vi "Enqueue Power Spectrum.vi"(6 "plot analys?":bool, 7 "plot data?":bool, 8 "error in (no error)":errorcluster, 9 "pwr spctm":cluster{"f0":dbl, "df":dbl, "magnitude":dbl[]}, 10 "wfm dat":waveform(cdb), 11 "plot queue":refnum<queue>) -> (0 "error out":errorcluster)   [LabVIEW 2021]
uses:
  Plotting Data.ctl
  Plotting Message.ctl
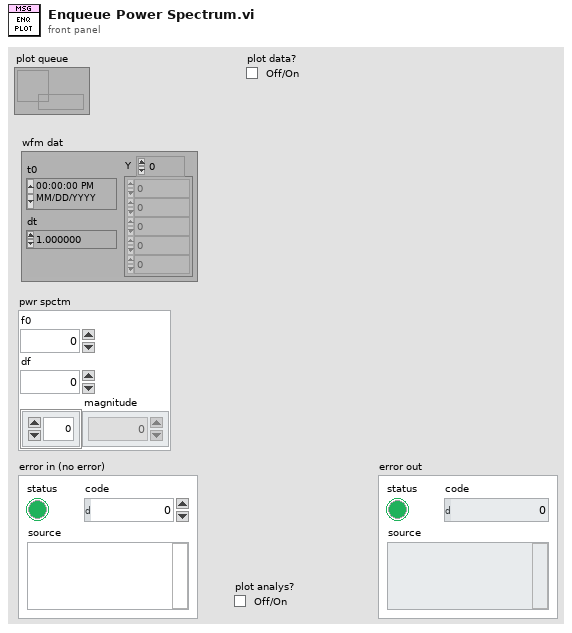
[diagram p1: front panel]
types:
  T1 = typedef "Plotting Data.ctl" = cluster{"wfm dat":waveform(cdb), "pwr sptm":cluster{"f0":dbl, "df":dbl, "magnitude":dbl[]}, "msg":T2}
  T2 = typedef "Plotting Message.ctl" = enum16{"Plot Anlalyzed Data", "Plot Acquired Data", "Exit"}
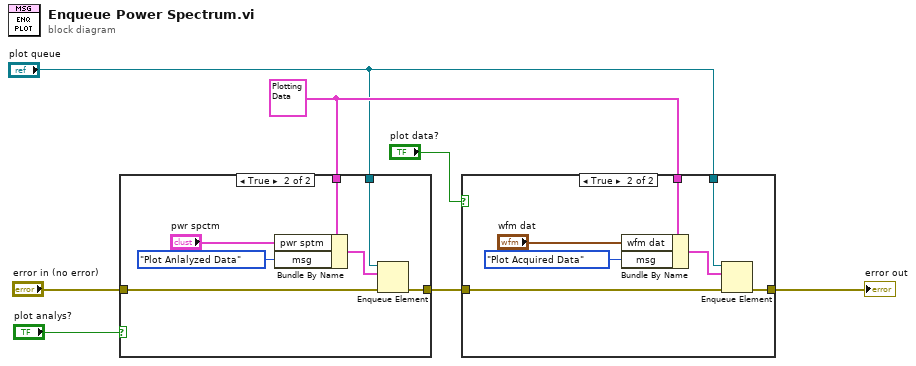
[diagram p0: block diagram]
diagram:
  w3 = T1 {"wfm dat"={"t0"=timestamp(0 s since 1904-01-01), "dt"=0.0, "Y"=[]}, "pwr sptm"={"f0"=0.0, "df"=0.0, "magnitude"=[]}, "msg"=enum."Plot Anlalyzed Data"} ("element")
  n1 = case shown="True" "plot analys?" {
    tunnel: [w8 w15] -> w4
    tunnel: "error in (no error)" -> [w8 w14]
    tunnel: "plot queue" -> [_ w13]
    tunnel: w3 -> [_ w12]
    frame False {
    }
    frame True {
      n2 = Bundle By Name(cluster=w12, "pwr sptm"="pwr spctm", "msg"=Plotting_Message."Plot Anlalyzed Data") -> (w10:T1)
      n3 = Enqueue Element(queue=w13, element=w10, error in (no error)=w14) -> (error out=w15:errorcluster)  [unwired: 1 in, 2 out]
    }
  }
  n4 = case shown="True" "plot data?" {
    tunnel: [w16 w23] -> w5
    tunnel: w4 -> [w16 w22]
    tunnel: "plot queue" -> [_ w21]
    tunnel: w3 -> [_ w20]
    frame False {
    }
    frame True {
      n5 = Bundle By Name(cluster=w20, "wfm dat"="wfm dat", "msg"=Plotting_Message."Plot Acquired Data") -> (w18:T1)
      n6 = Enqueue Element(queue=w21, element=w18, error in (no error)=w22) -> (error out=w23:errorcluster)  [unwired: 1 in, 2 out]
    }
  }
  "error out" <- w5
